vi "Read 0mq-Tcp command.vi"(8 "error in (no error)":errorcluster, 11 "ICS in":refnum<class "ICS.lvclass">) -> (0 "error out":errorcluster, 1 "isAcommand":bool, 2 "command":string, 3 "ICS out":refnum<class "ICS.lvclass">, 4 "rec0mq":bool)   [LabVIEW 2018, in "ICS.lvclass"]
uses:
  ICS.lvclass
  ICS.lvclass/ICS.ctl
  TCP-Server/TCP-Server.lvclass
  Messenger/Messenger.lvclass
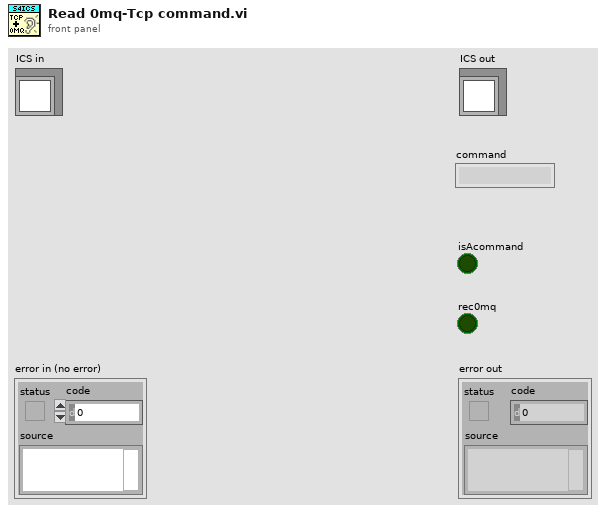
[diagram p1: front panel]
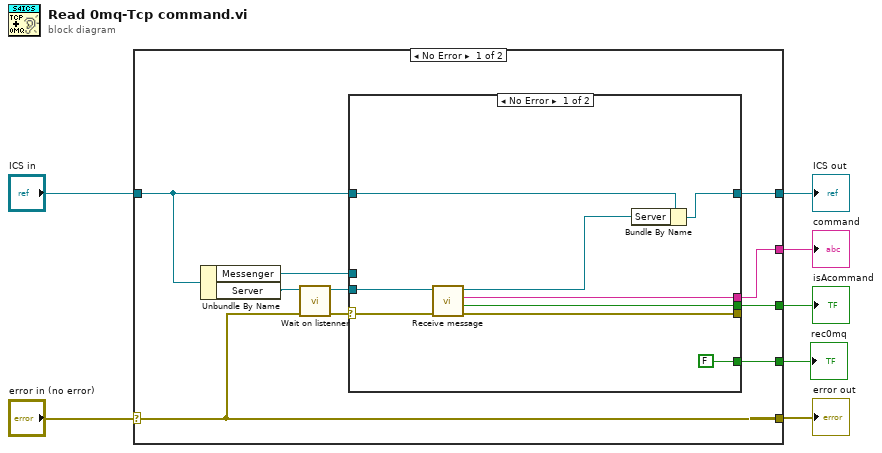
[diagram p0: block diagram]
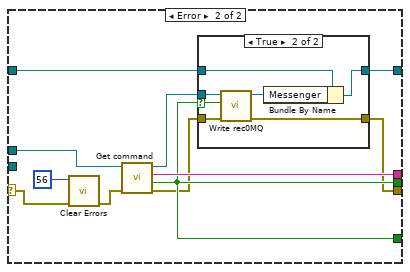
[diagram p2: hidden frame]
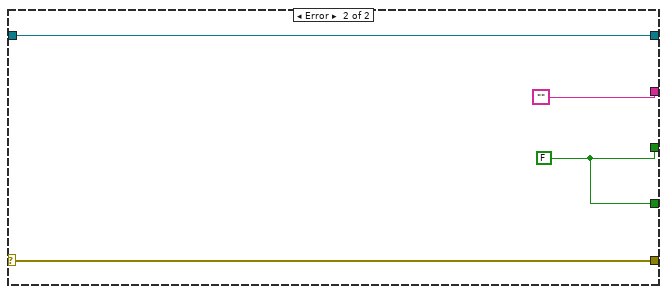
[diagram p4: hidden frame]
diagram:
  n1 = case shown="No Error" "error in (no error)" {
    selector: "error in (no error)" -> [w14 w50]
    tunnel: [w14 w50] -> w6
    tunnel: [w13 w49] -> w4
    tunnel: "ICS in" -> [w12 w49]
    tunnel: [w10 w47] -> w2
    tunnel: [w9 ""] -> w3
    tunnel: [w8 w47] -> w1
    frame No Error {
      n2 = Unbundle By Name(w12) -> ("Messenger"=w11:refnum<class "Messenger.lvclass">, "Server"=w16:refnum<class "TCP-Server.lvclass">)
      n3 = call-dynamic "Wait on listenner.vi"("error in (no error)"=w14, "Server in"=w16) -> ("error out"=w15:errorcluster, "Server out"=w17:refnum<class "TCP-Server.lvclass">)  [unwired: 8 in]
      n4 = case shown="No Error" w15 {
        selector: w15 -> [w26 w36]
        tunnel: w17 -> [w22 _]
        tunnel: [w25 w27] -> _
        tunnel: [w23 w30] -> w10
        tunnel: [w24 w33] -> w9
        tunnel: [w20 w31] -> w13
        tunnel: w12 -> [w21 w32]
        tunnel: w11 -> [_ w35]
        tunnel: [FALSE w30] -> w8
        frame No Error {
          n5 = call-dynamic "Receive message.vi"("error in (no error)"=w26, "Server in"=w22) -> ("error out"=w25:errorcluster, "isAcommand"=w23:bool, "message"=w24:string, "Server out"=w19:refnum<class "TCP-Server.lvclass">)  [unwired: 6 in]
          n6 = Bundle By Name(cluster=w21, "Server"=w19) -> (w20:refnum<class "ICS.lvclass">)
        }
        frame Error {
          n7 = call <vilib>:"Clear Errors.vi"("error in (no error)"=w36, "specific error code to clear (0: all)"=56) -> ("error out"=w34:errorcluster)  [unwired: 4 in, 1 out]
          n8 = call-dynamic "Get command.vi"("error in (no error)"=w34, "Messenger in"=w35) -> ("error out"=w28:errorcluster, "isAcommand"=w30:bool, "command"=w33:string, "Messenger out"=w29:refnum<class "Messenger.lvclass">)  [unwired: 6 in]
          n9 = case shown="True" w30 {
            selector: w30 -> [_ w40]
            tunnel: w32 -> [w39 w46]
            tunnel: [w39 w45] -> w31
            tunnel: w29 -> [_ w43]
            tunnel: w28 -> [w38 w42]
            tunnel: [w38 w41] -> w27
            frame False {
            }
            frame True {
              n10 = call-dynamic "Write rec0MQ.vi"("error in (no error)"=w42, "rec0MQ"=w40, "Messenger in"=w43) -> ("error out"=w41:errorcluster, "Messenger out"=w44:refnum<class "Messenger.lvclass">)  [unwired: 7 in]
              n11 = Bundle By Name(cluster=w46, "Messenger"=w44) -> (w45:refnum<class "ICS.lvclass">)
            }
          }
        }
      }
    }
    frame Error {
      w47 = FALSE
    }
  }
  "error out" <- w6
  "ICS out" <- w4
  "isAcommand" <- w2
  "command" <- w3
  "rec0mq" <- w1
